vi "Get Chars.vi"(7 "Scrollback":refnum<class "TermBuffer.lvclass">, 8 "error in (no error)":errorcluster, 10 "Start (Beginning)":i32, 11 "TermBuffer in":refnum<class "TermBuffer.lvclass">) -> (0 "error out":errorcluster, 2 "TermChars":T1[][](array[typedef]), 3 "TermBuffer out":refnum<class "TermBuffer.lvclass">)   [LabVIEW 2020, in "Terminal.lvlib" / "TermBuffer.lvclass"]
doc: "Provides a 2D array of <b>TermChars</b> based on the requested region.\n\n<b>Start</b> is intended to be 0 or negative. If <b>Start</b> is negative then lines from that far back will pulled from the provided scrollback buffer, if available. The number of rows and columns will be based on the currently configured buffer dimensions."
uses:
  TermBuffer.lvclass
  Term Char.ctl
  TermBuffer.lvclass/TermBuffer.ctl
  TermLine/TermLine.lvclass
  Terminal.lvlib
  Text Attributes.ctl
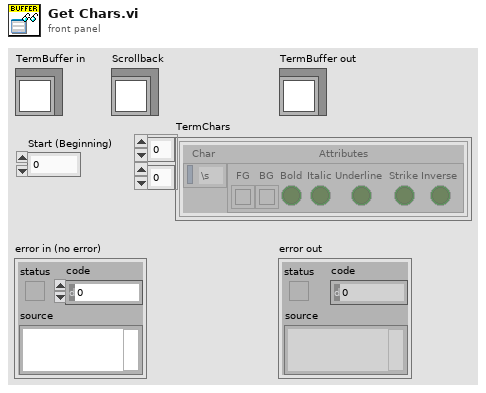
[diagram p1: front panel]
types:
  T1 = typedef "Terminal.lvlib/Term Char.ctl" = cluster{"Char":string, "Attributes":T2}
  T2 = typedef "Terminal.lvlib/Text Attributes.ctl" = cluster{"FG":u32, "BG":u32, "Bold":bool, "Italic":bool, "Underline":bool, "Strike":bool, "Inverse":bool}
  T3 = typedef "Terminal.lvlib/TermBuffer.lvclass/Ref Data.ctl" = cluster{"Lines":refnum<class "TermLine.lvclass">[], "Rows":i32, "Cols":i32}
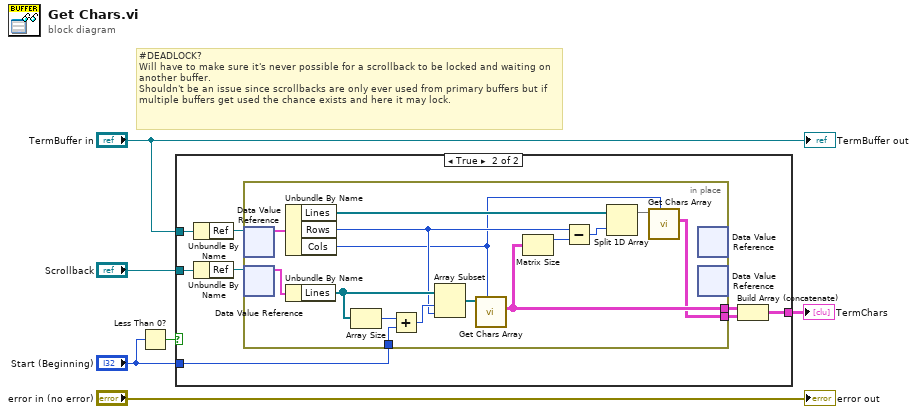
[diagram p0: block diagram]
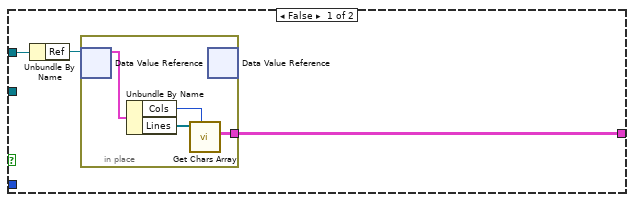
[diagram p2: hidden frame]
diagram:
  # "#DEADLOCK?\nWill have to make sure it's never possible for a scrollback to be locked and waiting on another buffer.\nShouldn't be an issue since scrollbacks are only ever used from primary buffers but if multiple buffers get used the chance exists and here it may lock."
  n1 = Less Than 0?(x="Start (Beginning)") -> (x < 0?=w4:bool)
  n2 = case shown="True" w4 {
    tunnel: "Start (Beginning)" -> [_ w19]
    tunnel: "Scrollback" -> [_ w20]
    tunnel: [w7 w17] -> w2
    tunnel: "TermBuffer in" -> [w8 w15]
    frame False {
      n3 = Unbundle By Name(w8) -> ("Ref"=w9:refnum<data-value>)
      n4 = in-place {
        in-place-border: [w10] -> w7
        n5 = in-place-dvr #1(w9) -> (w13:T3)  [unwired: 1 out]
        n6 = Unbundle By Name(w13) -> ("Cols"=w11:i32, "Lines"=w12:refnum<class "TermLine.lvclass">[])
        n7 = call "Get Chars Array.vi"("Width"=w11, "Lines"=w12) -> ("TermChars"=w10:T1[][])  [unwired: 8 in, 1 out]
        n8 = in-place-dvr #1() -> ()  [unwired: 1 in, 2 out]
      }
    }
    frame True {
      n9 = Unbundle By Name(w15) -> ("Ref"=w16:refnum<data-value>)
      n10 = Unbundle By Name(w20) -> ("Ref"=w21:refnum<data-value>)
      n11 = in-place {
        in-place-border: w19 -> [w35]
        in-place-border: [w28] -> w18
        in-place-border: [w23] -> w14
        n12 = in-place-dvr #2(w16) -> (w31:T3)  [unwired: 1 out]
        n13 = in-place-dvr #3(w21) -> (w36:T3)  [unwired: 1 out]
        n14 = Unbundle By Name(w31) -> ("Lines"=w27:refnum<class "TermLine.lvclass">[], "Rows"=w26:i32, "Cols"=w24:i32)
        n15 = Unbundle By Name(w36) -> ("Lines"=w34:refnum<class "TermLine.lvclass">[])
        n16 = Array Size(array=w34) -> (size(s)=w22:i32)
        n17 = Add(x=w22, y=w35) -> (x+y=w33:i32)
        n18 = Array Subset(array=w34, index=w33, length=w26) -> (w32:refnum<class "TermLine.lvclass">[])
        n19 = call "Get Chars Array.vi"("Width"=w24, "Lines"=w32) -> ("TermChars"=w28:T1[][])  [unwired: 8 in, 1 out]
        n20 = Matrix Size(0:w28) -> (1:w29:i32)  [unwired: 1 out]
        n21 = Subtract(x=w26, y=w29) -> (x-y=w30:i32)
        n22 = Split 1D Array(array=w27, index=w30) -> (first subarray=w25:refnum<class "TermLine.lvclass">[])  [unwired: 1 out]
        n23 = call "Get Chars Array.vi"("Width"=w24, "Lines"=w25) -> ("TermChars"=w23:T1[][])  [unwired: 8 in, 1 out]
        n24 = in-place-dvr #2() -> ()  [unwired: 1 in, 2 out]
        n25 = in-place-dvr #3() -> ()  [unwired: 1 in, 2 out]
      }
      n26 = Build Array (concatenate)(w18, w14) -> (w17:T1[][])
    }
  }
  "TermChars" <- w2
  "error out" <- "error in (no error)"
  "TermBuffer out" <- "TermBuffer in"
